vi "Number to Match.vi"() -> ()   [LabVIEW 2025]
uses:
  <vilib>/numeric/Random Number (Range) DBL.vi
panel:
  in  "stop":bool
  out "Iteration Count":i32
  in  "Number to Match":dbl min=0.0 max=100.0 step=1.0
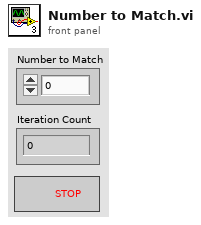
[diagram p1: front panel]
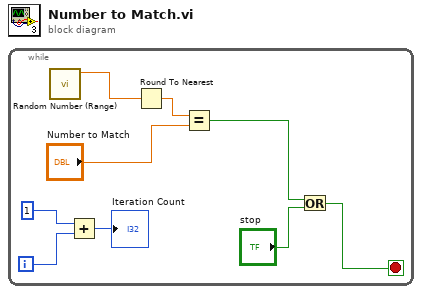
[diagram p0: block diagram]
diagram:
  n1 = while {
    i -> [w9]
    stop <- w1 stop-if-true
    n2 = call-poly <vilib>:"Random Number (Range).vi"() -> ("number"=w5:dbl)  [unwired: 11 in]
    n3 = Add(x=1, y=w9) -> (x+y=→"Iteration Count":i32)
    n4 = Round To Nearest(number=w5) -> (nearest integer value=w4:dbl)
    n5 = Equal?(x=w4, y="Number to Match") -> (x = y?=w2:bool)
    n6 = Or(x=w2, y="stop") -> (x .or. y?=w1:bool)
  }
